vi "Read Measurements.vi"(0 "VISA resource name":refnum<visa-resource-name>, 5 "error in (no error)":errorcluster) -> (8 "Current":dbl format="%_6f", 9 "Current Pk-Pk":dbl format="%_5g", 10 "Current Max":dbl format="%_5g", 11 "Power":dbl format="%_6f", 12 "Current Min":dbl format="%_6f", 13 "Resistance":dbl format="%_5g", 14 "VISA resource name out":refnum<visa-resource-name>, 15 "Voltage (V)":dbl format="%_6f", 16 "Voltage Max":dbl format="%_6f", 17 "Voltage Min":dbl format="%_6f", 18 "Voltage Pk-Pk":dbl format="%_5g", 19 "error out":errorcluster)   [LabVIEW 2019, in "BK Precision 8500B Series.lvlib"]
doc: "Measures several types of voltage and current parameters(level, max, min, pk-pk). The signal-oriented measurement commands are used to acquire readings. The user can use these high level instructions to control the measurement process."
uses:
  <instrlib>/BK Precision 8500B Series/BK Precision 8500B Series.lvlib
panel:
  # "V"
  # "V"
  # "V"
  # "V"
  # "A"
  # "A"
  # "V"
  # "A"
  # "V"
  # "A"
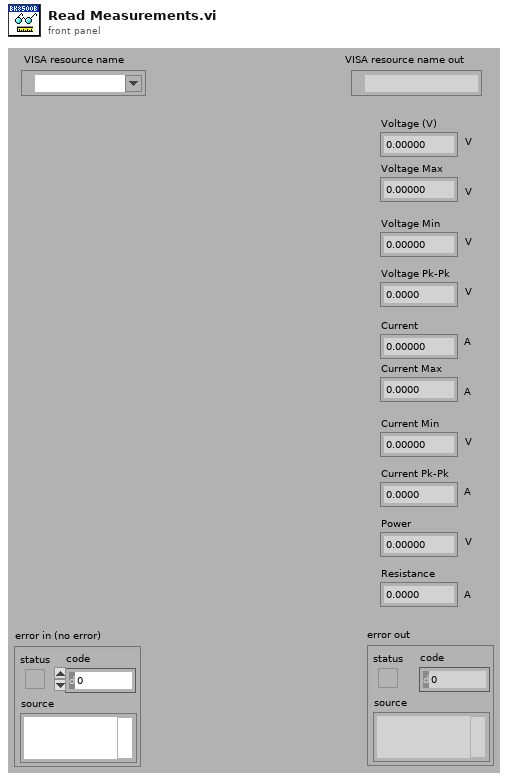
[diagram p1: front panel]
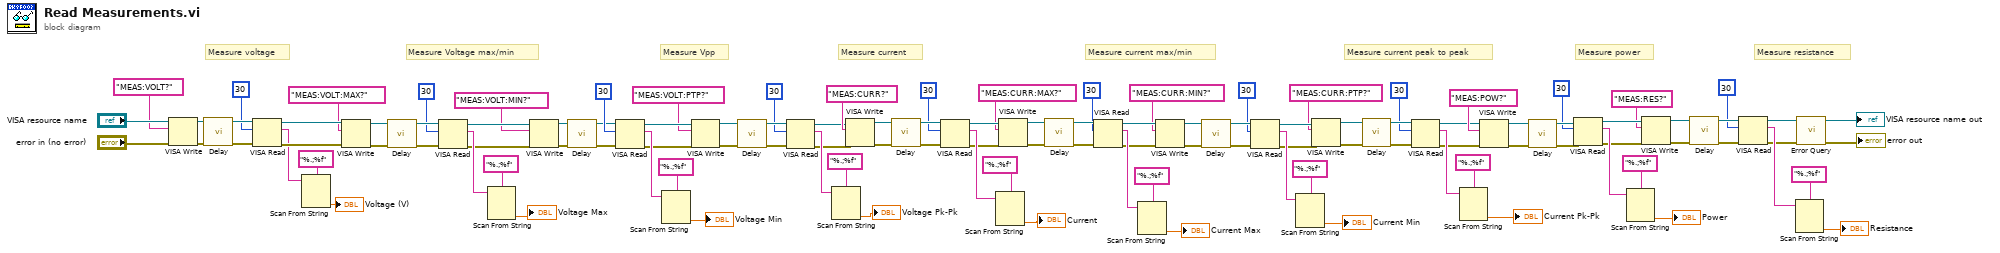
[diagram p0: block diagram]
diagram:
  # "Measure resistance"
  # "Measure power"
  # "Measure current peak to peak"
  # "Measure current max/min"
  # "Measure current"
  # "Measure Vpp"
  # "Measure Voltage max/min"
  # "Measure voltage"
  n1 = VISA Write(VISA resource name="VISA resource name", write buffer="MEAS:VOLT?", error in (no error)="error in (no error)") -> (VISA resource name out=w110:refnum<visa-resource-name>, error out=w108:errorcluster)  [unwired: 1 out]
  n2 = call <instrlib>:"Delay.vi"("error in (no error)"=w108, "VISA resource name"=w110) -> ("error out"=w107:errorcluster, "VISA resource name out"=w109:refnum<visa-resource-name>)  [unwired: 8 in]
  n3 = VISA Read(VISA resource name=w109, byte count=30, error in (no error)=w107) -> (VISA resource name out=w106:refnum<visa-resource-name>, read buffer=w97:string, error out=w105:errorcluster)  [unwired: 1 out]
  n4 = Scan From String(format string="%.;%f", input string=w97) -> (output 1=→"Voltage (V)":dbl)  [unwired: 3 in, 3 out]
  n5 = VISA Write(VISA resource name=w106, write buffer="MEAS:VOLT:MAX?", error in (no error)=w105) -> (VISA resource name out=w104:refnum<visa-resource-name>, error out=w103:errorcluster)  [unwired: 1 out]
  n6 = call <instrlib>:"Delay.vi"("error in (no error)"=w103, "VISA resource name"=w104) -> ("error out"=w101:errorcluster, "VISA resource name out"=w102:refnum<visa-resource-name>)  [unwired: 8 in]
  n7 = VISA Read(VISA resource name=w102, byte count=30, error in (no error)=w101) -> (VISA resource name out=w93:refnum<visa-resource-name>, read buffer=w95:string, error out=w92:errorcluster)  [unwired: 1 out]
  n8 = Scan From String(format string="%.;%f", input string=w95) -> (output 1=→"Voltage Max":dbl)  [unwired: 3 in, 3 out]
  n9 = VISA Write(VISA resource name=w93, write buffer="MEAS:VOLT:MIN?", error in (no error)=w92) -> (VISA resource name out=w90:refnum<visa-resource-name>, error out=w89:errorcluster)  [unwired: 1 out]
  n10 = call <instrlib>:"Delay.vi"("error in (no error)"=w89, "VISA resource name"=w90) -> ("error out"=w86:errorcluster, "VISA resource name out"=w87:refnum<visa-resource-name>)  [unwired: 8 in]
  n11 = VISA Read(VISA resource name=w87, byte count=30, error in (no error)=w86) -> (VISA resource name out=w69:refnum<visa-resource-name>, read buffer=w85:string, error out=w68:errorcluster)  [unwired: 1 out]
  n12 = Scan From String(format string="%.;%f", input string=w85) -> (output 1=→"Voltage Min":dbl)  [unwired: 3 in, 3 out]
  n13 = VISA Write(VISA resource name=w69, write buffer="MEAS:VOLT:PTP?", error in (no error)=w68) -> (VISA resource name out=w76:refnum<visa-resource-name>, error out=w74:errorcluster)  [unwired: 1 out]
  n14 = call <instrlib>:"Delay.vi"("error in (no error)"=w74, "VISA resource name"=w76) -> ("error out"=w73:errorcluster, "VISA resource name out"=w75:refnum<visa-resource-name>)  [unwired: 8 in]
  n15 = VISA Read(VISA resource name=w75, byte count=30, error in (no error)=w73) -> (VISA resource name out=w57:refnum<visa-resource-name>, read buffer=w72:string, error out=w56:errorcluster)  [unwired: 1 out]
  n16 = Scan From String(format string="%.;%f", input string=w72) -> (output 1=→"Voltage Pk-Pk":dbl)  [unwired: 3 in, 3 out]
  n17 = VISA Write(VISA resource name=w57, write buffer="MEAS:CURR?", error in (no error)=w56) -> (VISA resource name out=w65:refnum<visa-resource-name>, error out=w63:errorcluster)  [unwired: 1 out]
  n18 = call <instrlib>:"Delay.vi"("error in (no error)"=w63, "VISA resource name"=w65) -> ("error out"=w62:errorcluster, "VISA resource name out"=w64:refnum<visa-resource-name>)  [unwired: 8 in]
  n19 = VISA Read(VISA resource name=w64, byte count=30, error in (no error)=w62) -> (VISA resource name out=w47:refnum<visa-resource-name>, read buffer=w61:string, error out=w46:errorcluster)  [unwired: 1 out]
  n20 = Scan From String(format string="%.;%f", input string=w61) -> (output 1=→"Current":dbl)  [unwired: 3 in, 3 out]
  n21 = VISA Write(VISA resource name=w47, write buffer="MEAS:CURR:MAX?", error in (no error)=w46) -> (VISA resource name out=w54:refnum<visa-resource-name>, error out=w52:errorcluster)  [unwired: 1 out]
  n22 = call <instrlib>:"Delay.vi"("error in (no error)"=w52, "VISA resource name"=w54) -> ("error out"=w51:errorcluster, "VISA resource name out"=w53:refnum<visa-resource-name>)  [unwired: 8 in]
  n23 = VISA Read(VISA resource name=w53, byte count=30, error in (no error)=w51) -> (VISA resource name out=w34:refnum<visa-resource-name>, read buffer=w50:string, error out=w33:errorcluster)  [unwired: 1 out]
  n24 = Scan From String(format string="%.;%f", input string=w50) -> (output 1=→"Current Max":dbl)  [unwired: 3 in, 3 out]
  n25 = VISA Write(VISA resource name=w34, write buffer="MEAS:CURR:MIN?", error in (no error)=w33) -> (VISA resource name out=w41:refnum<visa-resource-name>, error out=w39:errorcluster)  [unwired: 1 out]
  n26 = call <instrlib>:"Delay.vi"("error in (no error)"=w39, "VISA resource name"=w41) -> ("error out"=w38:errorcluster, "VISA resource name out"=w40:refnum<visa-resource-name>)  [unwired: 8 in]
  n27 = VISA Read(VISA resource name=w40, byte count=30, error in (no error)=w38) -> (VISA resource name out=w23:refnum<visa-resource-name>, read buffer=w37:string, error out=w22:errorcluster)  [unwired: 1 out]
  n28 = Scan From String(format string="%.;%f", input string=w37) -> (output 1=→"Current Min":dbl)  [unwired: 3 in, 3 out]
  n29 = VISA Write(VISA resource name=w23, write buffer="MEAS:CURR:PTP?", error in (no error)=w22) -> (VISA resource name out=w30:refnum<visa-resource-name>, error out=w28:errorcluster)  [unwired: 1 out]
  n30 = call <instrlib>:"Delay.vi"("error in (no error)"=w28, "VISA resource name"=w30) -> ("error out"=w27:errorcluster, "VISA resource name out"=w29:refnum<visa-resource-name>)  [unwired: 8 in]
  n31 = VISA Read(VISA resource name=w29, byte count=30, error in (no error)=w27) -> (VISA resource name out=w13:refnum<visa-resource-name>, read buffer=w26:string, error out=w12:errorcluster)  [unwired: 1 out]
  n32 = Scan From String(format string="%.;%f", input string=w26) -> (output 1=→"Current Pk-Pk":dbl)  [unwired: 3 in, 3 out]
  n33 = VISA Write(VISA resource name=w13, write buffer="MEAS:POW?", error in (no error)=w12) -> (VISA resource name out=w83:refnum<visa-resource-name>, error out=w81:errorcluster)  [unwired: 1 out]
  n34 = call <instrlib>:"Delay.vi"("error in (no error)"=w81, "VISA resource name"=w83) -> ("error out"=w80:errorcluster, "VISA resource name out"=w82:refnum<visa-resource-name>)  [unwired: 8 in]
  n35 = VISA Read(VISA resource name=w82, byte count=30, error in (no error)=w80) -> (VISA resource name out=w11:refnum<visa-resource-name>, read buffer=w79:string, error out=w10:errorcluster)  [unwired: 1 out]
  n36 = Scan From String(format string="%.;%f", input string=w79) -> (output 1=→"Power":dbl)  [unwired: 3 in, 3 out]
  n37 = VISA Write(VISA resource name=w11, write buffer="MEAS:RES?", error in (no error)=w10) -> (VISA resource name out=w19:refnum<visa-resource-name>, error out=w9:errorcluster)  [unwired: 1 out]
  n38 = call <instrlib>:"Delay.vi"("error in (no error)"=w9, "VISA resource name"=w19) -> ("error out"=w8:errorcluster, "VISA resource name out"=w18:refnum<visa-resource-name>)  [unwired: 8 in]
  n39 = VISA Read(VISA resource name=w18, byte count=30, error in (no error)=w8) -> (VISA resource name out=w4:refnum<visa-resource-name>, read buffer=w17:string, error out=w3:errorcluster)  [unwired: 1 out]
  n40 = Scan From String(format string="%.;%f", input string=w17) -> (output 1=→"Resistance":dbl)  [unwired: 3 in, 3 out]
  n41 = call <instrlib>:"Error Query.vi"("error in (no error)"=w3, "VISA resource name"=w4) -> ("error out"=→"error out":errorcluster, "VISA resource name out"=→"VISA resource name out":refnum<visa-resource-name>)  [unwired: 6 in, 2 out]
